vi "Calibrate Potentiometers.vi"(8 "error in (no error)":errorcluster, 9 "rate":dbl=1000.0 format="%0.2f", 10 "DAQ  Channels In":T1={"Force Transducer: Left"="Dev1/ai6", "Force Transducer: Right "="Dev1/ai8", "EMG: Left"="", "EMG: Right"="", "Potentiometer: Left"="", "Potentiometer: Right"=""}, 11 "NI Force Task in":refnum<class "NI Force Task.lvclass">) -> (0 "error out":errorcluster, 3 "NI Force Task out":refnum<class "NI Force Task.lvclass">)   [LabVIEW 2020, in "NI Force Task.lvlib" / "NI Force Task.lvclass"]
uses:
  NI Force Task.lvclass
  NI Force Task.lvclass/NI Force Task.ctl
  <vilib>/DAQmx/create/channels.llb/DAQmx Create Channel (AI-Voltage-Basic).vi
  <vilib>/DAQmx/configure/timing.llb/DAQmx Timing (Sample Clock).vi
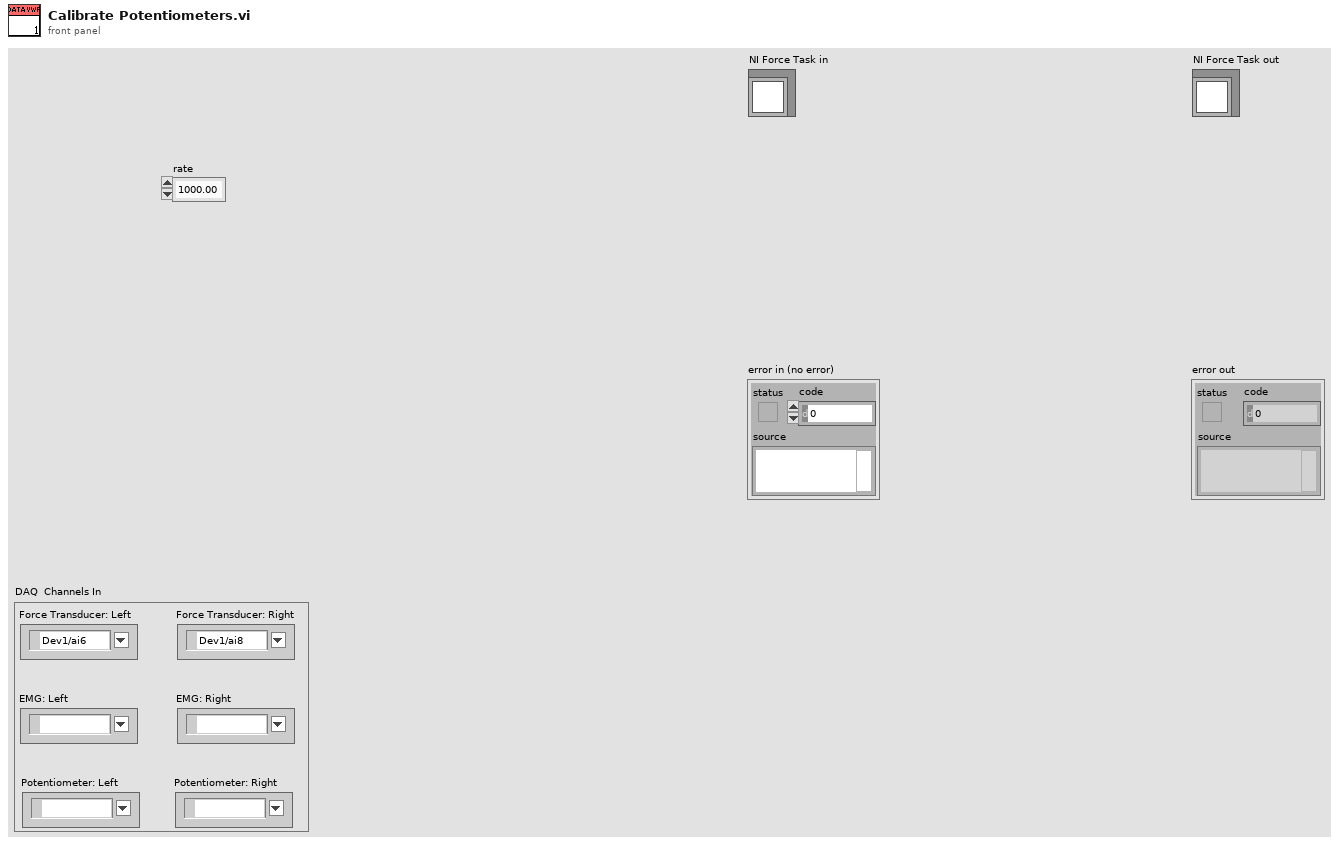
[diagram p1: front panel]
types:
  T1 = cluster{"Force Transducer: Left":tag, "Force Transducer: Right ":tag, "EMG: Left":tag, "EMG: Right":tag, "Potentiometer: Left":tag, "Potentiometer: Right":tag}
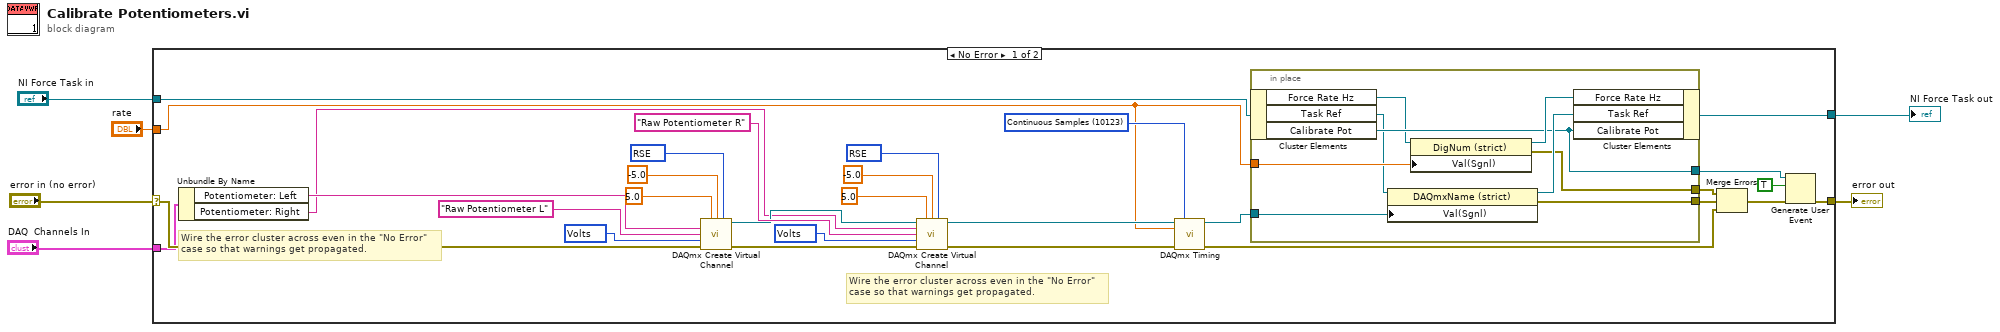
[diagram p0: block diagram]
diagram:
  n1 = case shown="No Error" "error in (no error)" {
    selector: "error in (no error)" -> [w10 w47]
    tunnel: [w11 w47] -> w5
    tunnel: [w12 w46] -> w3
    tunnel: "NI Force Task in" -> [w13 w46]
    tunnel: "rate" -> [w9 _]
    tunnel: "DAQ  Channels In" -> [w8 _]
    frame No Error {
      w22 = 10123 items=["Finite Samples"=10178, "Continuous Samples"=10123, "Hardware Timed Single Point"=12522] ("sample mode")
      w27 = 10348 items=["Volts"=10348, "From Custom Scale"=10065] ("units")
      w31 = 10083 items=["Default"=-1, "RSE"=10083, "NRSE"=10078, "Differential"=10106, "Pseudodifferential"=12529] ("input terminal configuration")
      w32 = 10348 items=["Volts"=10348, "From Custom Scale"=10065] ("units")
      w36 = 10083 items=["Default"=-1, "RSE"=10083, "NRSE"=10078, "Differential"=10106, "Pseudodifferential"=12529] ("input terminal configuration")
      # "Wire the error cluster across even in the \"No Error\"\ncase so that warnings get propagated."
      # "Wire the error cluster across even in the \"No Error\"\ncase so that warnings get propagated."
      n2 = Unbundle By Name(w8) -> ("Potentiometer: Left"=w24:tag, "Potentiometer: Right"=w23:tag)
      n3 = call-poly <vilib>:"DAQmx Create Virtual Channel.vi"("maximum value"=5.0, "minimum value"=-5.0, "input terminal configuration"=w36, "physical channels"=w24, "name to assign"="Raw Potentiometer L", "units"=w32, "error in"=w10) -> ("task out"=w26:refnum<k21>, "error out"=w25:errorcluster)  [unwired: 7 in]
      n4 = call-poly <vilib>:"DAQmx Create Virtual Channel.vi"("task in"=w26, "maximum value"=5.0, "minimum value"=-5.0, "input terminal configuration"=w31, "physical channels"=w23, "name to assign"="Raw Potentiometer R", "units"=w27, "error in"=w25) -> ("task out"=w21:refnum<k21>, "error out"=w20:errorcluster)  [unwired: 6 in]
      n5 = call-poly <vilib>:"DAQmx Timing.vi"("task/channels in"=w21, "sample mode"=w22, "rate"=w9, "error in"=w20) -> ("task out"=w19:refnum<k21>, "error out"=w16:errorcluster)  [unwired: 10 in]
      n6 = in-place {
        in-place-border: w9 -> [w43]
        in-place-border: w19 -> [w39]
        in-place-border: [w42] -> w18
        in-place-border: [w41] -> w17
        in-place-border: [w40] -> w7
        n7 = in-place-cluster #1(w13) -> ("Force Rate Hz"=w37:refnum<vi>, "Task Ref"=w38:refnum<vi>, "Calibrate Pot"=w40:refnum<user-event>)
        n8 = property class="DAQmxName (strict)"(reference=w38, "Val(Sgnl)"=w39) -> (reference out=w44:refnum<vi>, error out=w41:errorcluster)  [unwired: 1 in]
        n9 = property class="DigNum (strict)"(reference=w37, "Val(Sgnl)"=w43) -> (reference out=w45:refnum<vi>, error out=w42:errorcluster)  [unwired: 1 in]
        n10 = in-place-cluster #1("Force Rate Hz"=w45, "Task Ref"=w44, "Calibrate Pot"=w40) -> (w12:refnum<class "NI Force Task.lvclass">)
      }
      n11 = Merge Errors(w18, w17, w16) -> (w14:errorcluster)
      n12 = Generate User Event(user event=w7, event data cluster=TRUE ("event data"), error in=w14) -> (error out=w11:errorcluster)  [unwired: 1 in, 1 out]
    }
    frame Error {
    }
  }
  "error out" <- w5
  "NI Force Task out" <- w3
